vi "Swerve Motor Front Right.vi"(0 "Steer motor reference name":string="My Motor RefNum", 1 "Drive motor reference name":string="My Motor RefNum", 2 "Speed command":dbl, 3 "Direction command (deg)":dbl) -> ()   [LabVIEW 2018]
uses:
  <vilib>/Rock Robotics/WPI/ThirdParty/Phoenix-LabVIEW/Motor Controller/Controls/CTRE_Phoenix_MotorControl_ControlMode.ctl
  <vilib>/Rock Robotics/WPI/ThirdParty/Phoenix-LabVIEW/Motor Controller/Get/CTRE_Phoenix_MotorController_GetAnalogData.vi
  Robot Global Data.vi
  <vilib>/Rock Robotics/WPI/ThirdParty/REV Robotics/SPARK MAX/Typedef/Spark MAX Control Type.ctl
panel:
  out "s? t:f":dbl
  out "Veloicity":dbl
  out "Better Angle":dbl
  out "New Posiition":dbl
  out "Front Right Angle":dbl
  out "Position (Raw Sensor Units)":i32
  # "VI inputs"
  # "Intermediate values"
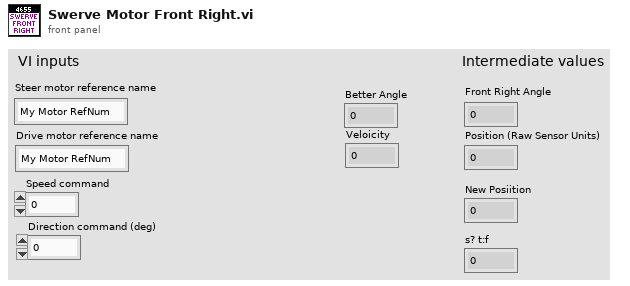
[diagram p1: front panel]
types:
  T1 = typedef "WPI_MotorControlDeviceRef.ctl" = cluster{"DeviceStatus":errorcluster, "Type":T2, "PWM":cluster{"PWM Channel":T3, "DeadBand":T4}, "CAN":cluster{"Device Number":u8, "SetOutput VI Ref":variant, "GetOutput VI Ref":variant, "Enable VI Ref":variant, "Disable VI Ref":variant, "Data":variant}, "Invert":bool, "DIO PWM":cluster{"PWM \"Enable\" Channel":T3, "DIOChannel":T5, "PWM Rate":dbl}}
  T2 = typedef "WPI_MotorControlType.ctl" = enum16{"PWM", "CAN", "DIO PWM"}
  T3 = typedef "FPGA_DIOPWMChannel.ctl" = enum8{"PWM 0", "PWM 1", "PWM 2", "PWM 3", "PWM 4", "PWM 5", "PWM 6", "PWM 7", "PWM 8", "PWM 9", "PWM MXP 0", "PWM MXP 1", "PWM MXP 2", "PWM MXP 3", "PWM MXP 4", "PWM MXP 5", "PWM MXP 6", "PWM MXP 7", "PWM MXP 8", "PWM MXP 9", "Invalid"}
  T4 = typedef "WPI_PWMDeadband.ctl" = cluster{"Name":string, "maxPositivePwm":i32, "minPositivePwm":i32, "centerPwm":i32, "maxNegativePwm":i32, "minNegativePwm":i32, "angularRange":u16}
  T5 = typedef "FPGA_DIOChannel.ctl" = enum8{"DIO 0", "DIO 1", "DIO 2", "DIO 3", "DIO 4", "DIO 5", "DIO 6", "DIO 7", "DIO 8", "DIO 9", "DIO MXP 0", "DIO MXP 1", "DIO MXP 2", "DIO MXP 3", "DIO MXP 4", "DIO MXP 5", "DIO MXP 6", "DIO MXP 7", "DIO MXP 8", "DIO MXP 9", "DIO MXP 10", "DIO MXP 11", "DIO MXP 12", "DIO MXP 13", "DIO MXP 14", "DIO MXP 15", "SPI Port CS1", "SPI Port CS2", "SPI Port CS3", "SPI Port MISO", "SPI Port MOSI", "Invalid"}
  T6 = typedef "CTRE_Phoenix_MotorControl_ControlMode.ctl" = u16
  T7 = typedef "Spark MAX Control Type.ctl" = enum16{"Percent VBus", "Voltage", "Velocity", "Position", "Smart Motion", "Current", "Smart Velocity"}
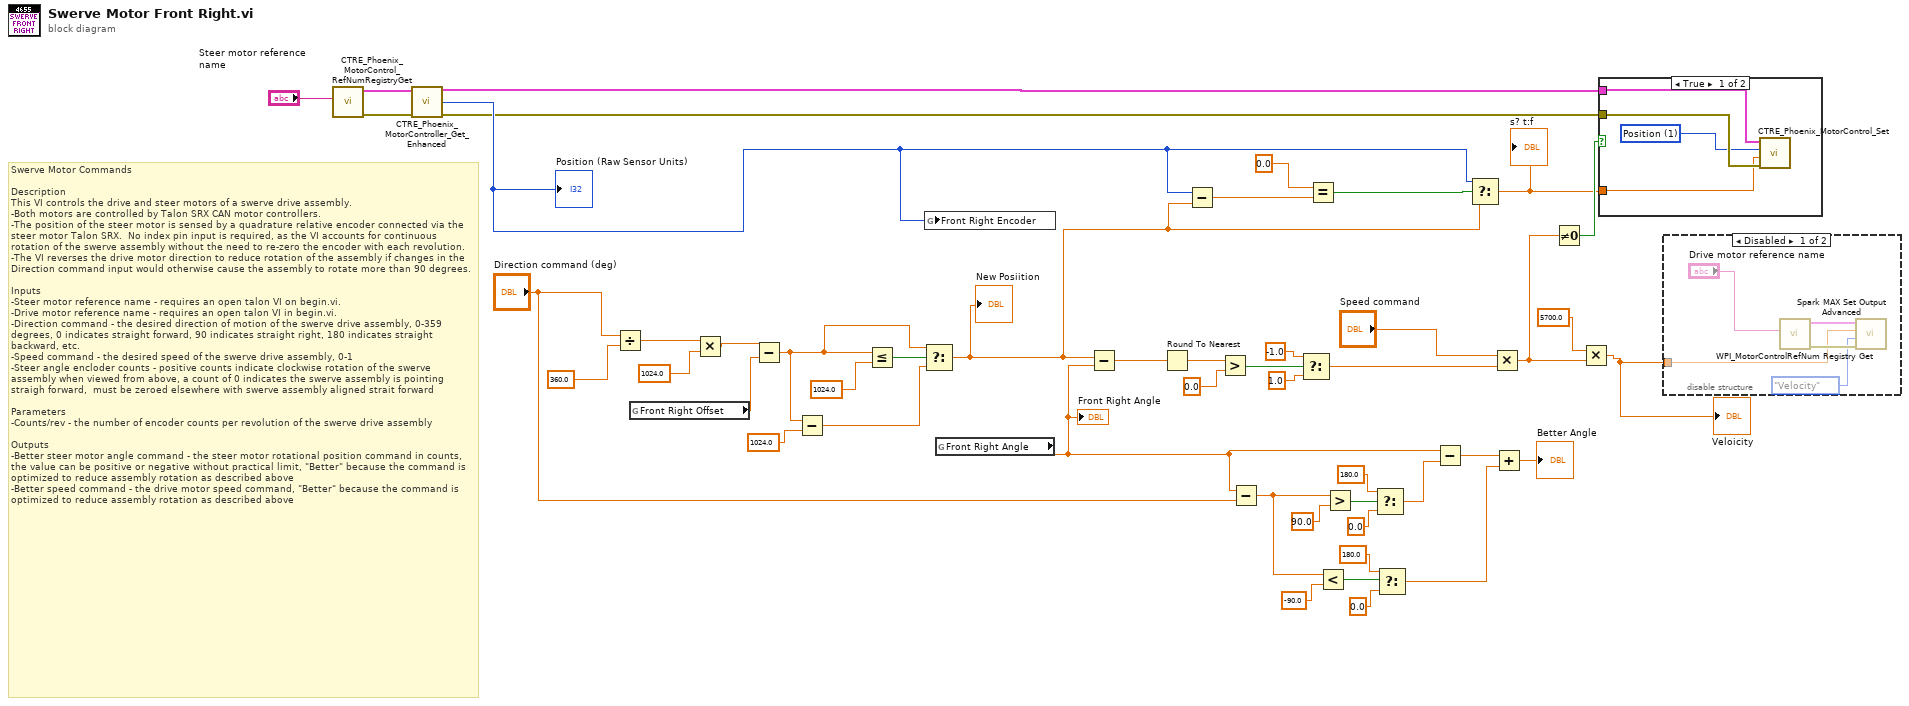
[diagram p0: block diagram]
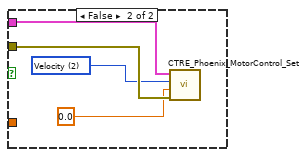
[diagram p3: hidden frame]
diagram:
  # "Swerve Motor Commands\n\nDescription\nThis VI controls the drive and steer motors of a swerve drive assembly.  \n-Both motors are controlled by Talon SRX CAN motor controllers.  \n-The position of the steer motor is sensed by a quadrature relative encoder connected via the steer motor Talon SRX.  No index pin input is required, as the VI accounts for continuous rotation of the swerve assembly without the need to re-zero the encoder with each revolution.\n-The VI reverses the drive motor direction to reduce rotation of the assembly if changes in the Direction command input would otherwise cause the assembly to rotate more than 90 degrees.\n\nInputs\n-Steer motor reference name - requires an open talon VI on begin.vi.\n-Drive motor reference name - requires an open talon VI in begin.vi.\n-Direction command - the desired direction of motion of the swerve drive assembly, 0-359 degrees, 0 indicates straight forward, 90 indicates straight right, 180 indicates straight backward, etc.\n-Speed command - the desired speed of the swerve drive assembly, 0-1\n-Steer angle encloder counts - positive counts indicate clockwise rotation of the swerve assembly when viewed from above, a count of 0 indicates the swerve assembly is pointing straigh forward,  must be zeroed elsewhere with swerve assembly aligned strait forward\n\nParameters\n-Counts/rev - the number of encoder counts per revolution of the swerve drive assembly\n\nOutputs\n-Better steer motor angle command - the steer motor rotational position command in counts, the value can be positive or negative without practical limit, \"Better\" because the command is optimized to reduce assembly rotation as described above\n-Better speed command - the drive motor speed command, \"Better\" because the command is optimized to reduce assembly rotation as described above"
  n1 = call <vilib>:"CTRE_Phoenix_MotorControl_RefNumRegistryGet.vi"("refnum name"="Steer motor reference name") -> ("error out"=w46:errorcluster, "PhoenixMotorControlDevRef"=w47:T1)  [unwired: 9 in]
  n2 = call-poly <vilib>:"CTRE_Phoenix_MotorController_Get_Enhanced.vi"("PhoenixMotorControlDevRef"=w47, "error in"=w46) -> ("PhoenixMotorControlDevRef"=w4:T1, "AnalogInRaw"=w9:i32, "error out"=w3:errorcluster)  [unwired: 9 in, 2 out]
  "Position (Raw Sensor Units)" <- w9
  n3 = Divide(x="Direction command (deg)", y=360.0 ("x*y")) -> (x/y=w36:dbl)
  n4 = global read "Robot Global Data.vi" "Front Right Offset"() -> (w33:dbl)
  n5 = Multiply(x=w36, y=1024.0 ("x")) -> (x*y=w34:dbl)
  n6 = Subtract(x=w34, y=w33) -> (x-y=w28:dbl)
  n7 = Subtract(x=w28, y=1024.0 ("x")) -> (x-y=w29:dbl)
  n8 = Less Or Equal?(x=w28, y=1024.0 ("x")) -> (x <= y?=w30:bool)
  n9 = Select(t=w28, s=w30, f=w29) -> (s? t:f=w8:dbl)
  "New Posiition" <- w8
  n10 = global write "Robot Global Data.vi" "Front Right Encoder"(w9) -> ()
  n11 = global read "Robot Global Data.vi" "Front Right Angle"() -> (w11:dbl)
  "Front Right Angle" <- w11
  n12 = Subtract(x=w8, y=w11) -> (x-y=w40:dbl)
  n13 = Round To Nearest(number=w40) -> (nearest integer value=w42:dbl)
  n14 = Subtract(x=w9, y=w8) -> (x-y=w10:dbl)
  n15 = Greater?(x=w42, y=0.0) -> (0:w39:bool)
  n16 = Subtract(x=w11, y="Direction command (deg)") -> (x-y=w16:dbl)
  n17 = Select(t=-1.0, s=w39, f=1.0) -> (s? t:f=w27:dbl)
  n18 = Equal?(x=0.0, y=w10) -> (x = y?=w38:bool)
  n19 = Less?(x=w16, y=-90.0) -> (x < y?=w18:bool)
  n20 = Greater?(x=w16, y=90.0) -> (0:w25:bool)
  n21 = Select(t=180.0, s=w25, f=0.0) -> (s? t:f=w21:dbl)
  n22 = Select(t=180.0, s=w18, f=0.0) -> (s? t:f=w14:dbl)
  n23 = Subtract(x=w11, y=w21) -> (x-y=w15:dbl)
  n24 = Select ("hold current steer angle\nif speed command is zero")(t=w9, s=w38, f=w8) -> (s? t:f=w2:dbl)
  "s? t:f" <- w2
  n25 = Multiply(x="Speed command", y=w27) -> (x*y=w1:dbl)
  n26 = Add(x=w15, y=w14) -> (x+y=→"Better Angle":dbl)
  n27 = Not Equal To 0?(x=w1) -> (x != 0?=w5:bool)
  n28 = Multiply(x=5700.0, y=w1) -> (x*y=w6:dbl)
  "Veloicity" <- w6
  n29 = case shown="True" w5 {
    tunnel: w4 -> [w52 w56]
    tunnel: w3 -> [w51 w55]
    tunnel: w2 -> [w50 _]
    frame True {
      w49 = T6 1 items=["PercentOutput"=0, "Position"=1, "Velocity"=2, "Current"=3, "Follower"=5, "MotionProfile"=6, "MotionMagic"=7, "MotionProfileArc"=10, "Disabled"=15] ("Control Mode")
      n30 = call <vilib>:"CTRE_Phoenix_MotorControl_Set.vi"("error in (no error)"=w51, "Output"=w50, "Control Mode"=w49, "PhoenixMotorControlDevRef"=w52) -> ()  [unwired: 6 in, 2 out]
    }
    frame False {
      w54 = T6 2 items=["PercentOutput"=0, "Position"=1, "Velocity"=2, "Current"=3, "Follower"=5, "MotionProfile"=6, "MotionMagic"=7, "MotionProfileArc"=10, "Disabled"=15] ("Control Mode")
      n31 = call <vilib>:"CTRE_Phoenix_MotorControl_Set.vi"("error in (no error)"=w55, "Output"=0.0 ("y"), "Control Mode"=w54, "PhoenixMotorControlDevRef"=w56) -> ()  [unwired: 6 in, 2 out]
    }
  }
  n32 = disable-structure shown="Disabled" {
    disable-tunnel: w6 -> [w57 _]
    frame Disabled {
      n33 = call <vilib>:"WPI_MotorControlRefNum Registry Get.vi"("refnum name"="Drive motor reference name") -> ("error out"=w61:errorcluster, "MotorControlDevRef"=w60:T1)  [unwired: 9 in]
      n34 = call <vilib>:"Spark MAX Set Output Advanced.vi"("error in (no error)"=w61, "Control Mode"=Spark_MAX_Control_Type."Velocity", "Setpoint"=w57, "MotorControlDevRef"=w60) -> ()  [unwired: 6 in, 2 out]
    }
    frame Enabled {
    }
  }
